vi "GUI PS Main Window.vi"() -> ()   [LabVIEW 2011]
uses:
  Types Definitions/Type GUI PS.ctl
  <vilib>/Platform/TimedLoop/XDataNode/timing_clust.ctl
  <vilib>/Platform/TimedLoop/XDataNode/nitl_modes.ctl
  <vilib>/Platform/TimedLoop/XDataNode/wakeup.ctl
  Types Definitions/Type Configuration Data (GUI to Controller).ctl
  Types Definitions/Type FOFB Parameters.ctl
  Types Definitions/Type Network Configuration.ctl
  Types Definitions/Type FA Configuration.ctl
  Types Definitions/Type Response Matrix Measurement Configuration.ctl
  Types Definitions/Type Correction Algorithm Configuration.ctl
  Types Definitions/Type Acquisition Network Configuration.ctl
  Types Definitions/Type Actuation Network Configuration.ctl
  Types Definitions/Type Configuration Change Acknowledge (Controller to GUI).ctl
  Types Definitions/Type TCP State.ctl
  <vilib>/Platform/TimedLoop/XDataNode/XDataNode.xnode
  <vilib>/Platform/TimedLoop/XDataNode/XDNodeRunTimeDep.lvlib
  LNLS Control VIs.lvlib
  Misc VIs.lvlib
  Type Definitions.lvlib
panel:
  out "PS Status":bool[](array[boolean])
  out "PS Setpoints":dbl[](array[numeric])
  in  "Step":dbl caption="Step (A)"
  in  "Configuration":dbl caption="Ajuste (A)"
  in  "Stop Test":bool
  out "Status":bool
  out "error out":errorcluster
  in  "PS Settings":bool
  in  "Initialize Test":bool
  # "FONTES CORRETORAS"
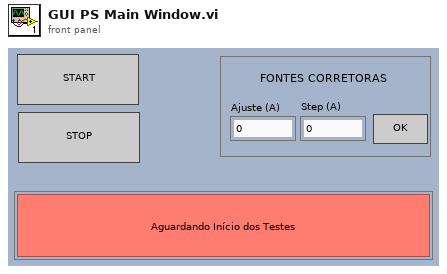
[diagram p1: front panel]
types:
  T1 = typedef "Type Definitions.lvlib/Type GUI PS.ctl" = cluster{"Change PS Value":refnum<notifier>, "Initialize/Stop RMM":refnum<notifier>, "Stop VI":refnum<notifier>, "Step Setpoint":refnum<notifier>}
  T2 = typedef "XDNodeRunTimeDep.lvlib/timing_clust.ctl" = cluster{"Expected End [f-1]":u64, "Actual End [f-1]":u64, "Finished Late? [f-1]":bool, "Expected End [i-1]":u64, "Actual End [i-1]":u64, "Finished Late? [i-1]":bool, "Expected Start [i]":u64, "Actual Start [i]":u64, "Expected Start [f]":u64, "Actual Start [f]":u64, "Source Name":string, "Structure Name":string, "Period":i64, "Deadline":i64, "Offset":i64, "Start":i64, "Priority":i32, "Timeout":i32, "Mode":T3, "Wakeup Reason":T4, "Error":errorcluster, "Source Type":string, "Secondary Source Type":string, "Global End Time":u64, "Global Start Time":u64, "Frame Duration":u64, "Iteration Duration":u64, "Assigned CPU":i32, "I/O Scan Engine Mode":u32}
  T3 = typedef "XDNodeRunTimeDep.lvlib/nitl_modes.ctl" = enum32{"No Change", "Process missed periods, maintain original phase", "Discard missed periods, maintain original phase", "Process missed periods, ignore original phase", "Discard missed periods, ignore original phase"}
  T4 = typedef "XDNodeRunTimeDep.lvlib/wakeup.ctl" = enum32{"Normal", "Aborted", "Asynchronous wakeup", "Timing source error", "Timed loop error", "Timeout"}
  T5 = enum16{"Wait Connection", "Read Data", "Write Data", "Close Connection", "Idle"}
  T6 = enum16{"Idle Mode", "Error Mode", "Manual Mode", "FOFB Mode", "RMM Mode"}
  T7 = cluster{"Operation Mode":enum16{"Idle Mode", "Error Mode", "Manual Mode", "FOFB Mode", "RMM Mode"}, "Correction Period (usec)":i32, "Beam Energy (MeV)":sgl, "Beam Current (mA)":sgl}
  T8 = typedef "Type Definitions.lvlib/Type LOCON_BIPOLAR_16BITS.ctl" = cluster{"priority":u8, "flag":u8, "analog value":u16, "status":u8}
  T9 = enum16{"Idle", "Wait Connection", "Read Data", "Process Data", "Write Data", "Close Connection"}
  T10 = typedef "Type Definitions.lvlib/Type Configuration Data (GUI to Controller).ctl" = cluster{"Update Controller Soft Configuration":bool[], "Request RT Execution Trace":string[], "Reference Orbit":dbl[], "Request Response Matrix Folder List":bool[], "Request FOFB Parameters":bool[], "FOFB Parameters":T11[]}
  T11 = typedef "Type Definitions.lvlib/Type FOFB Parameters.ctl" = cluster{"Network":T12, "Fast Acquisition":T13, "Response Matrix Measurement":T14, "Correction Algorithm":T15, "Acquisition Network":T16, "Actuation Network":T17}
  T12 = typedef "Type Definitions.lvlib/Type Network Configuration.ctl" = cluster{"FOFB Controller IP":string, "LNLS Control Network IP":string, "LNLS Control Network Power Supplies TCP Port":u16, "LNLS Control Network FOFB Configuration TCP Port":u16, "Data Server TCP Port":u16, "Monitoring Data TCP Port":u16, "Configuration GUI TCP Port":u16, "TCP Listening Timeout":i32}
  T13 = typedef "Type Definitions.lvlib/Type FA Configuration.ctl" = cluster{"Acquisition Period":u32, "Data Buffer Size":u32, "Monitoring Period":u32}
  T14 = typedef "Type Definitions.lvlib/Type Response Matrix Measurement Configuration.ctl" = cluster{"Step Amplitude":dbl, "Time Between Steps":u32, "Step Duration":u32, "Number of Averages":u32}
  T15 = typedef "Type Definitions.lvlib/Type Correction Algorithm Configuration.ctl" = cluster{"Correction Period":u32, "Reference Orbit Path":path, "Response Matrix Path":path, "Correction Matrix Path":path, "Horizontal Correction Factor":dbl, "Vertical Correction Factor":dbl, "Beam Current FOFB Threshold":dbl, "Decouple H-V":bool, "Use Additional BPM LPF":bool, "BPM LPF Cutoff":dbl}
  T16 = typedef "Type Definitions.lvlib/Type Acquisition Network Configuration.ctl" = cluster{"Chassis Name":string, "Variables":cluster{"Variable Name":string, "Matrix Order":u32, "Location":dbl, "Plane":enum8{"H", "V"}, "On Correction":bool}[]}[]
  T17 = typedef "Type Definitions.lvlib/Type Actuation Network Configuration.ctl" = cluster{"Chassis Name":string, "Variables":cluster{"Variable Name":string, "Matrix Order":u32, "RMM Step Factor":dbl, "Plane":enum8{"H", "V"}, "On Correction":bool, "Kc":dbl, "Ti":dbl, "Td":dbl}[]}[]
  T18 = typedef "Type Definitions.lvlib/Type Configuration Change Acknowledge (Controller to GUI).ctl" = cluster{"Request Response Matrix List Folder":string[], "FOFB Parameters":T11[]}
  T19 = typedef "Type Definitions.lvlib/Type TCP State.ctl" = enum16{"Idle", "Wait Connection", "Read Data", "Process Data", "Write Data", "Close Connection"}
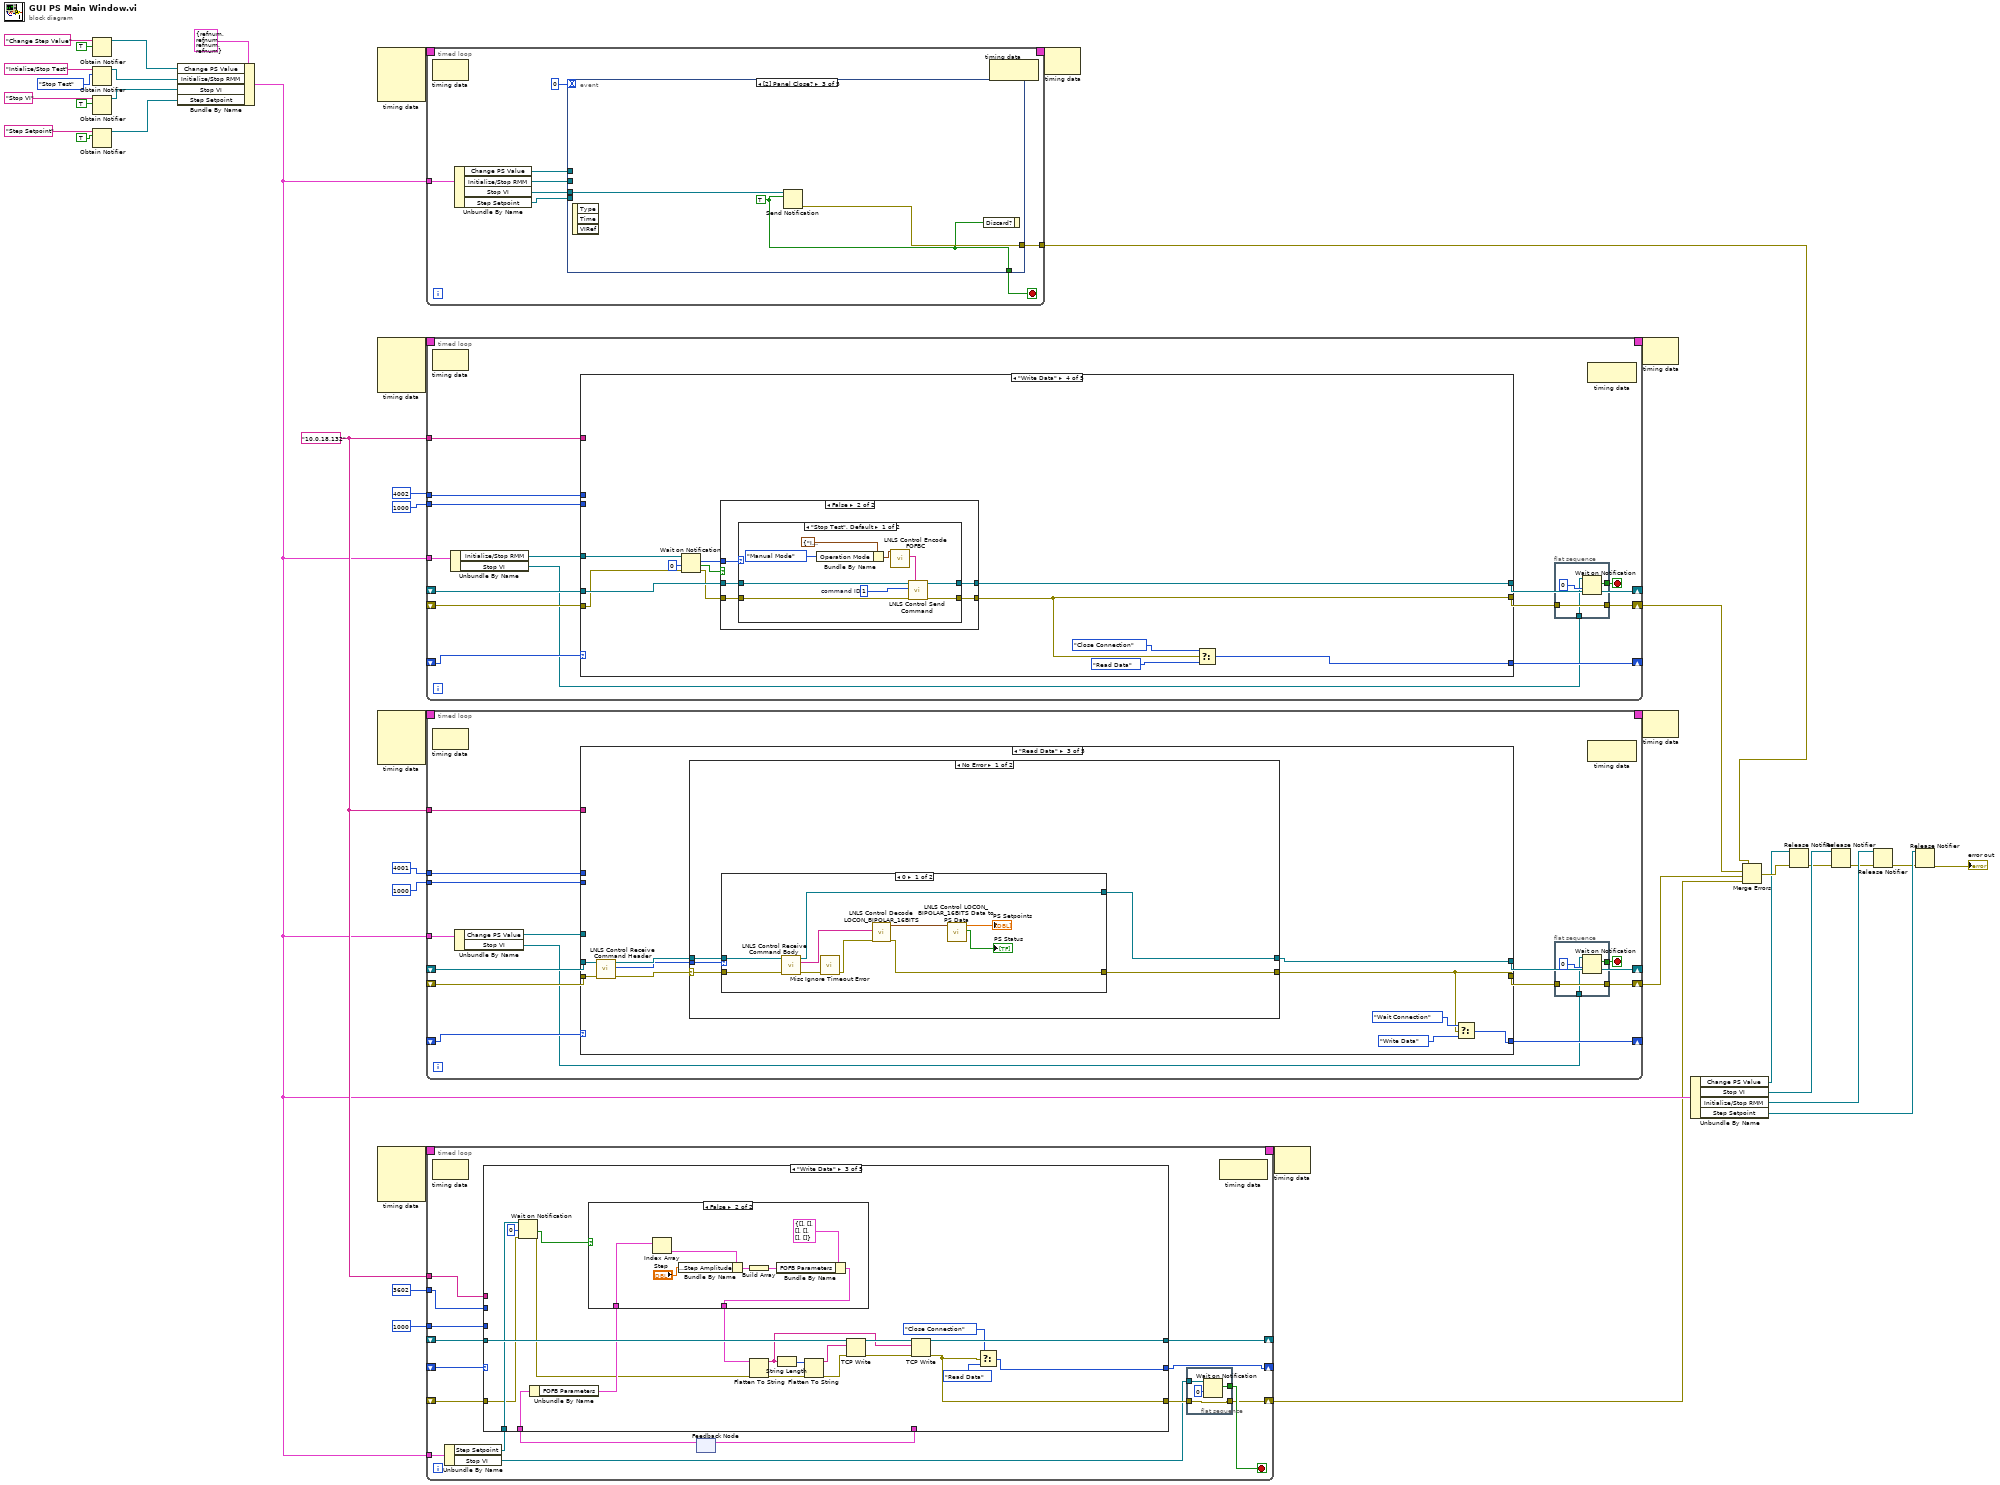
[diagram p0: block diagram]
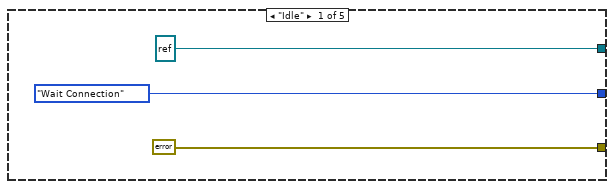
[diagram p2: hidden frame]
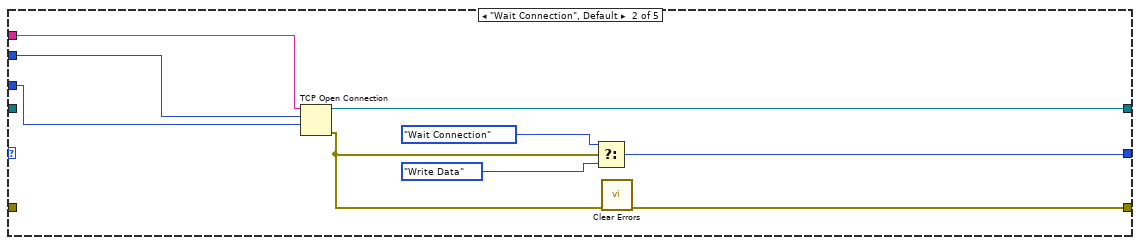
[diagram p3: hidden frame]
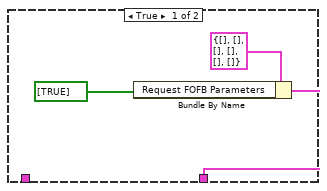
[diagram p4: hidden frame]
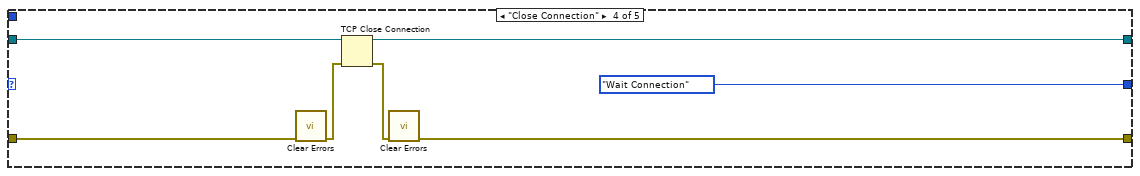
[diagram p5: hidden frame]
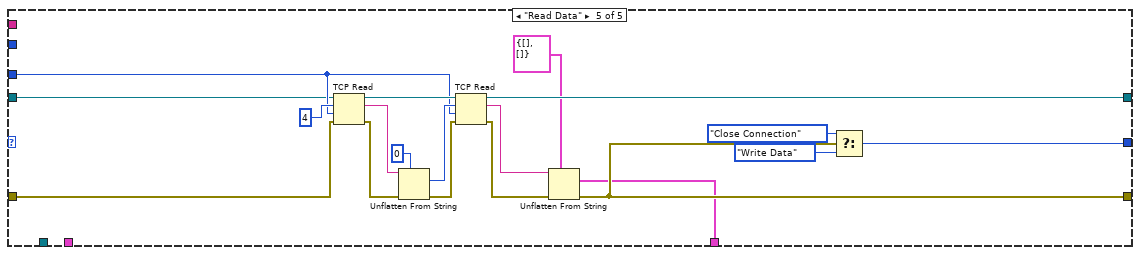
[diagram p6: hidden frame]
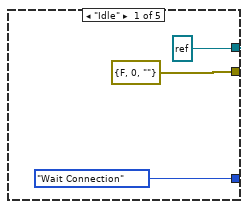
[diagram p7: hidden frame]
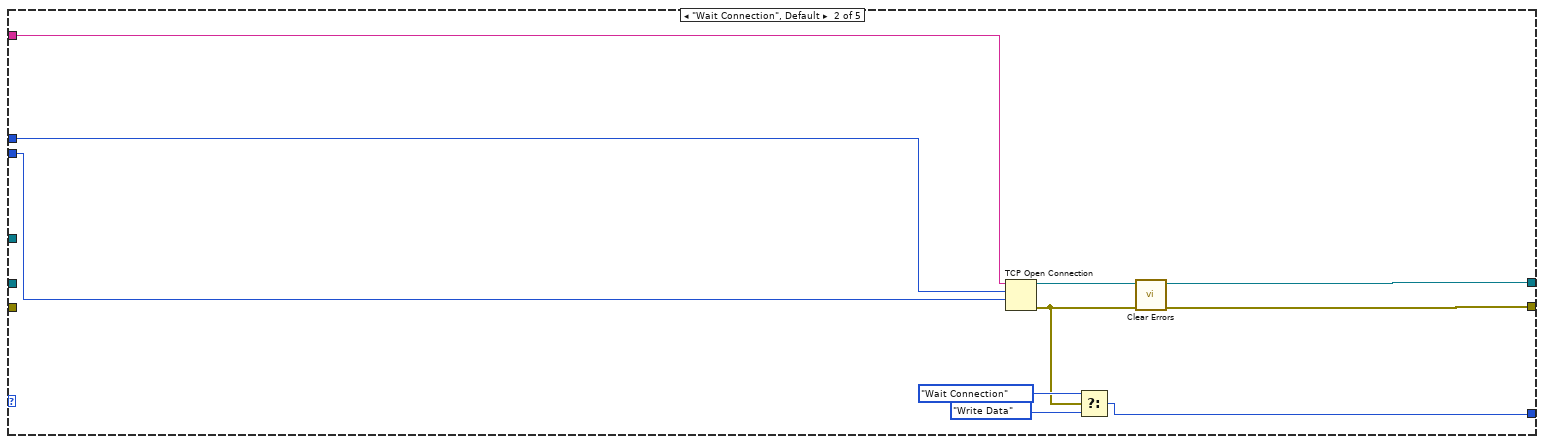
[diagram p8: hidden frame]
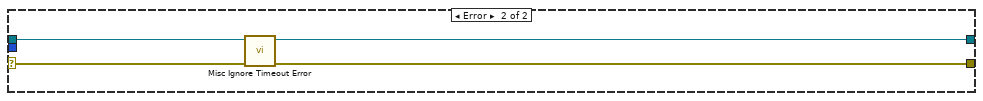
[diagram p10: hidden frame]
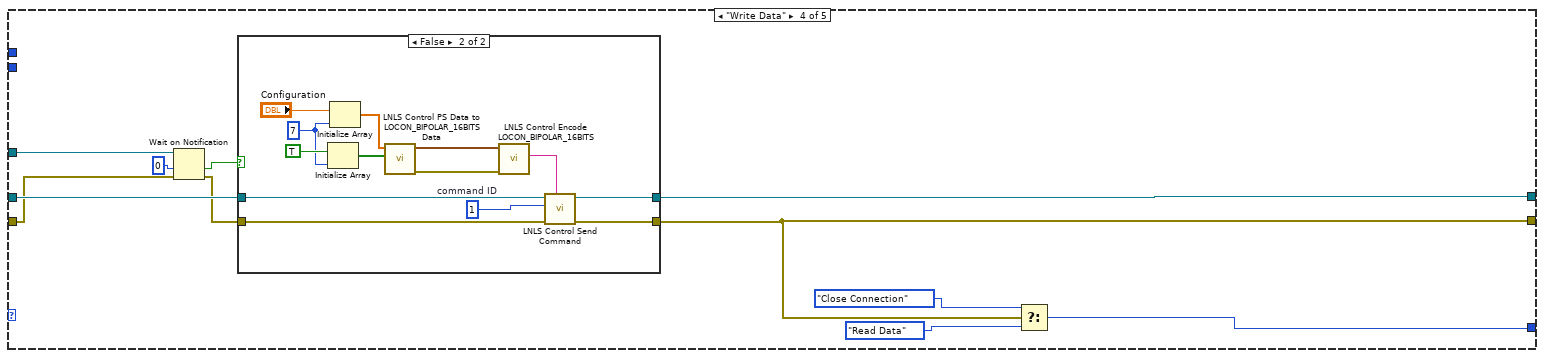
[diagram p11: hidden frame]
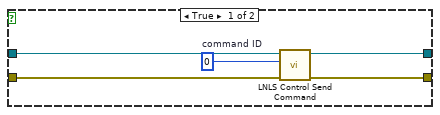
[diagram p12: hidden frame]
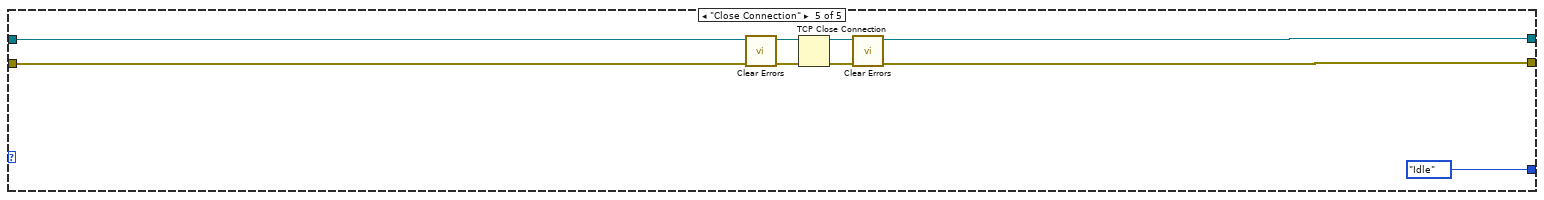
[diagram p13: hidden frame]
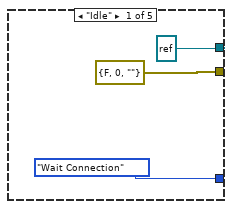
[diagram p14: hidden frame]
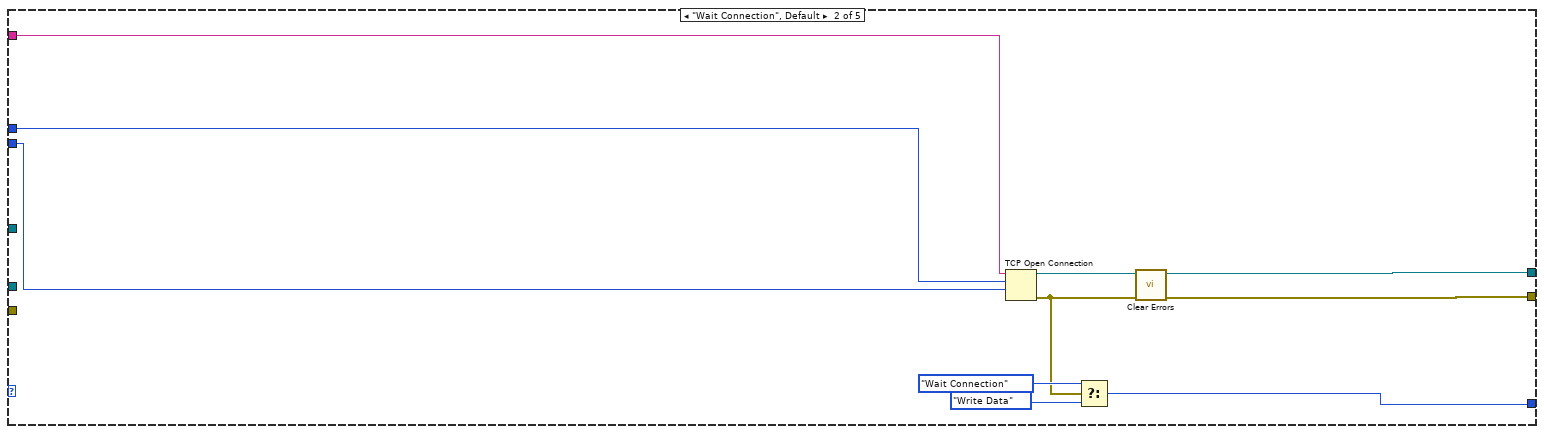
[diagram p15: hidden frame]
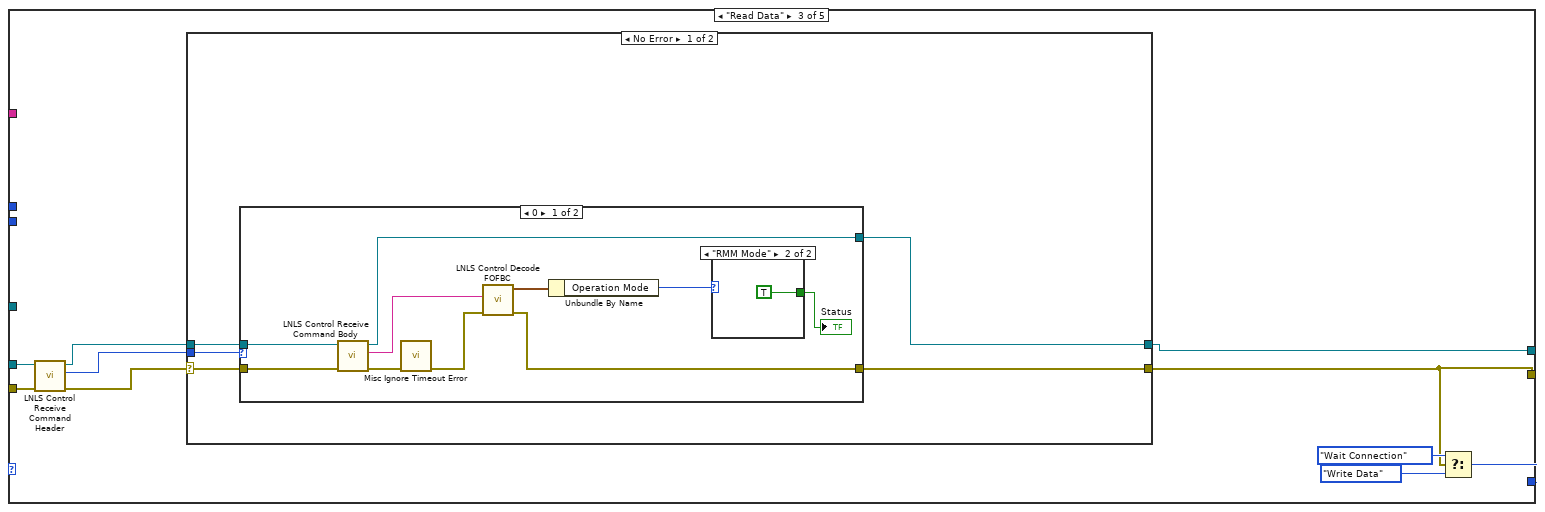
[diagram p16: hidden frame]
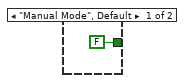
[diagram p17: hidden frame]
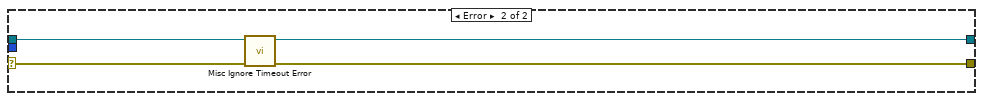
[diagram p19: hidden frame]
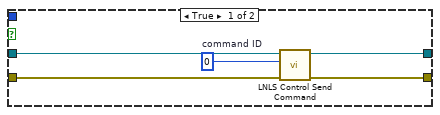
[diagram p20: hidden frame]
diagram:
  w12 = "10.0.18.132" ("address")
  n1 = Obtain Notifier(name (unnamed)="Change Step Value", notification data type=TRUE) -> (notifier out=w33:refnum<notifier>)  [unwired: 2 in, 2 out]
  n2 = Obtain Notifier(name (unnamed)="Intialize/Stop Test", notification data type=enum16{"Initialize Test", "Stop Test"}."Stop Test") -> (notifier out=w21:refnum<notifier>)  [unwired: 2 in, 2 out]
  n3 = Obtain Notifier(name (unnamed)="Stop VI", notification data type=TRUE) -> (notifier out=w32:refnum<notifier>)  [unwired: 2 in, 2 out]
  n4 = Obtain Notifier(name (unnamed)="Step Setpoint", notification data type=TRUE) -> (notifier out=w7:refnum<notifier>)  [unwired: 2 in, 2 out]
  n5 = Bundle By Name(cluster=T1 {"Change PS Value"=refnum, "Initialize/Stop RMM"=refnum, "Stop VI"=refnum, "Step Setpoint"=refnum} ("GUI PS"), "Change PS Value"=w33, "Initialize/Stop RMM"=w21, "Stop VI"=w32, "Step Setpoint"=w7) -> (w6:T1)
  n6 = node-c288() -> (w37:T2)  [unwired: 4 in]
  n7 = node-c288() -> (w26:T2)  [unwired: 4 in]
  n8 = node-c288() -> (w18:T2)  [unwired: 4 in]
  n9 = node-c288() -> (w14:T2)  [unwired: 4 in]
  n10 = timed-loop {
    timing: w37 -> [_]
    timing-out: [_] -> w36
    tunnel: [w48] -> w35
    tunnel: w6 -> [w47]
    stop <- w50 stop-if-true
    n11 = node-c288() -> ()  [unwired: 1 in, 1 out]
    n12 = Unbundle By Name(w47) -> ("Change PS Value"=w46:refnum<notifier>, "Initialize/Stop RMM"=w45:refnum<notifier>, "Stop VI"=w44:refnum<notifier>, "Step Setpoint"=w43:refnum<notifier>)
    n13 = event shown="[2] Panel Close?" {
      selector: _ -> [_ _ _ _ _]
      dyn-events: _ -> [_ _ _ _ _]
      timeout: 0 -> [_ _ _ _ _]
      tunnel: [_ _ w55 _ _] -> w50
      tunnel: [_ _ w57 _ _] -> w48
      tunnel: w46 -> [_ _ _ _ w64]
      tunnel: w45 -> [_ w52 _ w59 _]
      tunnel: w44 -> [_ _ w56 _ _]
      tunnel: w43 -> [_ _ _ _ w62]
      event Timeout {
        n14 = event-data() -> ()  [unwired: 1 in, 2 out]
      }
      event "Stop Test": Value Change {
        n15 = event-data() -> ("NewVal"=w51:bool)  [unwired: 1 in, 4 out]
        n16 = case shown="True" w51 {
          tunnel: w52 -> [_ w54]
          frame False {
          }
          frame True {
            n17 = Send Notification(notification=enum16{"Initialize Test", "Stop Test"}."Stop Test", notifier=w54) -> ()  [unwired: 1 in, 2 out]
          }
        }
      }
      event Panel Close? {
        w55 = TRUE
        n18 = event-data() -> ()  [unwired: 1 in, 3 out]
        n19 = Send Notification(notification=w55, notifier=w56) -> (error out=w57:errorcluster)  [unwired: 1 in, 1 out]
        n20 = event-data("Discard?"=w55) -> ()  [unwired: 1 in, 1 out]
      }
      event "Initialize Test": Value Change {
        n21 = event-data() -> ("NewVal"=w58:bool)  [unwired: 1 in, 4 out]
        n22 = case shown="True" w58 {
          tunnel: w59 -> [_ w61]
          frame False {
          }
          frame True {
            n23 = Send Notification(notification=enum16{"Initialize Test", "Stop Test"}."Initialize Test", notifier=w61) -> ()  [unwired: 1 in, 2 out]
          }
        }
      }
      event "PS Settings": Value Change {
        n24 = event-data() -> ("NewVal"=w63:bool)  [unwired: 1 in, 4 out]
        n25 = case shown="True" w63 {
          selector: w63 -> [_ w65]
          tunnel: w64 -> [_ w67]
          tunnel: w62 -> [_ w66]
          frame False {
          }
          frame True {
            n26 = Send Notification(notification=w65, notifier=w67) -> ()  [unwired: 1 in, 2 out]
            n27 = Send Notification(notification=w65, notifier=w66) -> ()  [unwired: 1 in, 2 out]
          }
        }
      }
    }
    n28 = node-c288() -> ()  [unwired: 1 in, 1 out]
  }
  n29 = timed-loop {
    shift-right: [w81] -> _
    shift-left: _ -> [w83]
    shift-right: [w82] -> _
    shift-left: _ -> [w80]
    shift-right: [w74] -> w20
    shift-left: _ -> [w79]
    tunnel: u16 4002 ("remote port or service name") -> [w78]
    tunnel: 1000 ("timeout ms (60000)") -> [w76]
    timing: w26 -> [_]
    timing-out: [_] -> w25
    tunnel: w12 -> [w73]
    tunnel: w6 -> [w72]
    stop <- w77 stop-if-true
    n30 = node-c288() -> ()  [unwired: 1 in, 1 out]
    n31 = Unbundle By Name(w72) -> ("Initialize/Stop RMM"=w70:refnum<notifier>, "Stop VI"=w71:refnum<notifier>)
    n32 = case shown="\"Write Data\"" w83 {
      tunnel: [refnum<k5> refnum ("connection ID") w94 w107 w137 w175] -> w82
      tunnel: [errorcluster {"status"=FALSE, "code"=0, "source"=""} ("error out") w92 w99 w139 w172] -> w75
      tunnel: [T5."Wait Connection" w97 w106 w140 T5."Idle"] -> w81
      tunnel: w80 -> [_ _ w104 w138 w176]
      tunnel: w79 -> [_ _ w105 w133 w170]
      tunnel: w78 -> [_ w91 _ _ _]
      tunnel: w76 -> [_ w90 _ _ _]
      tunnel: w73 -> [_ w89 _ _ _]
      tunnel: w70 -> [_ _ _ w136 _]
      frame "Idle" {
      }
      frame "Wait Connection", Default {
        n33 = TCP Open Connection(address=w89, remote port or service name=w91, timeout ms (60000)=w90) -> (connection ID=w94:refnum<k5>, error out=w93:errorcluster)  [unwired: 2 in]
        n34 = Select(t=T5."Wait Connection", s=w93, f=T5."Write Data") -> (s? t:f=w97:T5)
        n35 = call <vilib>:"Clear Errors.vi"("error in (no error)"=w93) -> ("error out"=w92:errorcluster)  [unwired: 6 in]
      }
      frame "Read Data" {
        n36 = call "LNLS Control Receive Command Header.vi"("error in (no error)"=w105, "connection ID"=w104) -> ("error out"=w101:errorcluster, "command ID"=w98:u8, "connection ID out"=w103:refnum<k5>)  [unwired: 7 in]
        n37 = case shown="No Error" w101 {
          selector: w101 -> [w111 w128]
          tunnel: [w110 w129] -> w107
          tunnel: [w108 w127] -> w99
          tunnel: w103 -> [w112 w129]
          tunnel: w98 -> [w109 _]
          frame No Error {
            n38 = case shown="0" w109 {
              tunnel: w112 -> [w122 w126]
              tunnel: w111 -> [w121 w125]
              tunnel: [w120 w126] -> w110
              tunnel: [w119 w125] -> w108
              frame 0 {
                n39 = call "LNLS Control Receive Command Body.vi"("error in (no error)"=w121, "connection ID"=w122) -> ("error out"=w118:errorcluster, "command body"=w116:string, "connection ID out"=w120:refnum<k5>)  [unwired: 6 in, 1 out]
                n40 = call "Misc Ignore Timeout Error.vi"("error in (no error)"=w118) -> ("error out"=w117:errorcluster)  [unwired: 10 in]
                n41 = call "LNLS Control Decode FOFBC.vi"("error in (no error)"=w117, "command body"=w116) -> ("error out"=w119:errorcluster, "LNLS Control FOFB Configuration"=w115:T7)  [unwired: 8 in]
                n42 = Unbundle By Name(w115) -> ("Operation Mode"=w114:T6)
                n43 = case shown="\"RMM Mode\"" w114 {
                  tunnel: [FALSE TRUE] -> w113
                  frame "Manual Mode", Default {
                  }
                  frame "RMM Mode" {
                  }
                }
                "Status" <- w113
              }
              frame 1, Default {
              }
            }
          }
          frame Error {
            n44 = call "Misc Ignore Timeout Error.vi"("error in (no error)"=w128) -> ("error out"=w127:errorcluster)  [unwired: 10 in]
          }
        }
        n45 = Select(t=T5."Wait Connection", s=w99, f=T5."Write Data") -> (s? t:f=w106:T5)
      }
      frame "Write Data" {
        n46 = Wait on Notification(notifier=w136, timeout in ms (-1)=0, error in (no error)=w133) -> (notification=w135:enum16{"Initialize Test", "Stop Test"}, timed out?=w130:bool, error out=w132:errorcluster)  [unwired: 1 in, 1 out]
        n47 = case shown="False" w130 {
          tunnel: [w144 w151] -> w139
          tunnel: w138 -> [w143 w150]
          tunnel: [w142 w149] -> w137
          tunnel: w135 -> [_ w148]
          tunnel: w132 -> [w145 w147]
          frame True {
            w146 = u8 0  # command ID
            n48 = call "LNLS Control Send Command.vi"("error in (no error)"=w145, "command ID"=w146, "connection ID"=w143) -> ("error out"=w144:errorcluster, "connection ID out"=w142:refnum<k5>)  [unwired: 7 in]
          }
          frame False {
            n49 = case shown="\"Stop Test\", Default" w148 {
              tunnel: w147 -> [w160 w169]
              tunnel: [w159 w168] -> w151
              tunnel: w150 -> [w158 w167]
              tunnel: [w157 w166] -> w149
              frame "Stop Test", Default {
                w156 = u8 1  # command ID
                n50 = Bundle By Name(cluster=T7 {"Operation Mode"=enum."Idle Mode", "Correction Period (usec)"=0, "Beam Energy (MeV)"=0.0, "Beam Current (mA)"=0.0} ("LNLS Control FOFB Configuration"), "Operation Mode"=T6."Manual Mode") -> (w152:T7)
                n51 = call "LNLS Control Encode FOFBC.vi"("LNLS Control FOFB Configuration"=w152) -> ("command body"=w155:string)  [unwired: 9 in, 1 out]
                n52 = call "LNLS Control Send Command.vi"("command body"=w155, "error in (no error)"=w160, "command ID"=w156, "connection ID"=w158) -> ("error out"=w159:errorcluster, "connection ID out"=w157:refnum<k5>)  [unwired: 6 in]
              }
              frame "Initialize Test" {
                w165 = u8 1  # command ID
                n53 = Bundle By Name(cluster=T7 {"Operation Mode"=enum."Idle Mode", "Correction Period (usec)"=0, "Beam Energy (MeV)"=0.0, "Beam Current (mA)"=0.0} ("LNLS Control FOFB Configuration"), "Operation Mode"=T6."RMM Mode") -> (w161:T7)
                n54 = call "LNLS Control Encode FOFBC.vi"("LNLS Control FOFB Configuration"=w161) -> ("command body"=w164:string)  [unwired: 9 in, 1 out]
                n55 = call "LNLS Control Send Command.vi"("command body"=w164, "error in (no error)"=w169, "command ID"=w165, "connection ID"=w167) -> ("error out"=w168:errorcluster, "connection ID out"=w166:refnum<k5>)  [unwired: 6 in]
              }
            }
          }
        }
        n56 = Select(t=T5."Close Connection", s=w139, f=T5."Read Data") -> (s? t:f=w140:T5)
      }
      frame "Close Connection" {
        n57 = call <vilib>:"Clear Errors.vi"("error in (no error)"=w170) -> ("error out"=w171:errorcluster)  [unwired: 6 in]
        n58 = TCP Close Connection(connection ID=w176, error in (no error)=w171) -> (connection ID out=w175:refnum<k5>, error out=w173:errorcluster)  [unwired: 1 in]
        n59 = call <vilib>:"Clear Errors.vi"("error in (no error)"=w173) -> ("error out"=w172:errorcluster)  [unwired: 6 in]
      }
    }
    n60 = flat-sequence {
      tunnel: [w179] -> w77
      tunnel: w75 -> [w178]
      tunnel: [w178] -> w74
      tunnel: w71 -> [w177]
      frame #0 {
        n61 = Wait on Notification(notifier=w177, timeout in ms (-1)=0) -> (notification=w179:bool)  [unwired: 2 in, 3 out]
      }
    }
    n62 = node-c288() -> ()  [unwired: 1 in, 1 out]
  }
  n63 = timed-loop {
    shift-right: [w192] -> _
    shift-left: _ -> [w194]
    shift-right: [w193] -> _
    shift-left: _ -> [w191]
    shift-right: [w185] -> w19
    shift-left: _ -> [w190]
    tunnel: u16 4001 ("remote port or service name") -> [w189]
    tunnel: 1000 ("timeout ms (60000)") -> [w187]
    timing: w18 -> [_]
    timing-out: [_] -> w17
    tunnel: w12 -> [w184]
    tunnel: w6 -> [w183]
    stop <- w188 stop-if-true
    n64 = node-c288() -> ()  [unwired: 1 in, 1 out]
    n65 = Unbundle By Name(w183) -> ("Change PS Value"=w181:refnum<notifier>, "Stop VI"=w182:refnum<notifier>)
    n66 = case shown="\"Read Data\"" w194 {
      tunnel: [refnum<k5> refnum ("connection ID") w205 w218 w245 w273] -> w193
      tunnel: [errorcluster {"status"=FALSE, "code"=0, "source"=""} ("error out") w203 w210 w247 w270] -> w186
      tunnel: [T5."Wait Connection" w208 w217 w248 T5."Idle"] -> w192
      tunnel: w191 -> [_ _ w215 w246 w274]
      tunnel: w190 -> [_ _ w216 w242 w268]
      tunnel: w189 -> [_ w202 _ _ _]
      tunnel: w187 -> [_ w201 _ _ _]
      tunnel: w184 -> [_ w200 _ _ _]
      tunnel: w181 -> [_ _ _ w244 _]
      frame "Idle" {
      }
      frame "Wait Connection", Default {
        n67 = TCP Open Connection(address=w200, remote port or service name=w202, timeout ms (60000)=w201) -> (connection ID=w205:refnum<k5>, error out=w204:errorcluster)  [unwired: 2 in]
        n68 = Select(t=T5."Wait Connection", s=w204, f=T5."Write Data") -> (s? t:f=w208:T5)
        n69 = call <vilib>:"Clear Errors.vi"("error in (no error)"=w204) -> ("error out"=w203:errorcluster)  [unwired: 6 in]
      }
      frame "Read Data" {
        n70 = call "LNLS Control Receive Command Header.vi"("error in (no error)"=w216, "connection ID"=w215) -> ("error out"=w212:errorcluster, "command ID"=w209:u8, "connection ID out"=w214:refnum<k5>)  [unwired: 7 in]
        n71 = case shown="No Error" w212 {
          selector: w212 -> [w222 w237]
          tunnel: [w221 w238] -> w218
          tunnel: [w219 w236] -> w210
          tunnel: w214 -> [w223 w238]
          tunnel: w209 -> [w220 _]
          frame No Error {
            n72 = case shown="0" w220 {
              tunnel: w223 -> [w233 w235]
              tunnel: w222 -> [w232 w234]
              tunnel: [w231 w235] -> w221
              tunnel: [w227 w234] -> w219
              frame 0 {
                n73 = call "LNLS Control Receive Command Body.vi"("error in (no error)"=w232, "connection ID"=w233) -> ("error out"=w230:errorcluster, "command body"=w229:string, "connection ID out"=w231:refnum<k5>)  [unwired: 6 in, 1 out]
                n74 = call "Misc Ignore Timeout Error.vi"("error in (no error)"=w230) -> ("error out"=w228:errorcluster)  [unwired: 10 in]
                n75 = call "LNLS Control Decode LOCON_BIPOLAR_16BITS.vi"("error in (no error)"=w228, "command body"=w229) -> ("error out"=w227:errorcluster, "LOCON data"=w226:T8[])  [unwired: 6 in]
                n76 = call "LNLS Control LOCON_BIPOLAR_16BITS Data to PS Data.vi"("PS Setpoints LOCON Data"=w226) -> ("PS Status"=→"PS Status":bool[], "PS Setpoints"=→"PS Setpoints":dbl[])  [unwired: 8 in, 1 out]
              }
              frame 1, Default {
              }
            }
          }
          frame Error {
            n77 = call "Misc Ignore Timeout Error.vi"("error in (no error)"=w237) -> ("error out"=w236:errorcluster)  [unwired: 10 in]
          }
        }
        n78 = Select(t=T5."Wait Connection", s=w210, f=T5."Write Data") -> (s? t:f=w217:T5)
      }
      frame "Write Data" {
        n79 = Wait on Notification(notifier=w244, timeout in ms (-1)=0, error in (no error)=w242) -> (timed out?=w239:bool, error out=w241:errorcluster)  [unwired: 1 in, 2 out]
        n80 = case shown="False" w239 {
          tunnel: [w252 w267] -> w247
          tunnel: w246 -> [w251 w266]
          tunnel: [w250 w265] -> w245
          tunnel: w241 -> [w253 w264]
          frame True {
            w254 = u8 0  # command ID
            n81 = call "LNLS Control Send Command.vi"("error in (no error)"=w253, "command ID"=w254, "connection ID"=w251) -> ("error out"=w252:errorcluster, "connection ID out"=w250:refnum<k5>)  [unwired: 7 in]
          }
          frame False {
            w256 = 7 ("dimension size")
            w263 = u8 1  # command ID
            n82 = Initialize Array(TRUE, w256) -> (w255:bool[])
            n83 = Initialize Array("Configuration", w256) -> (w258:dbl[])
            n84 = call "LNLS Control PS Data to LOCON_BIPOLAR_16BITS Data.vi"("PS Status"=w255, "PS Readings/Setpoints"=w258) -> ("error out"=w260:errorcluster, "PS Readings/Setpoints LOCON Data"=w262:T8[])  [unwired: 8 in]
            n85 = call "LNLS Control Encode LOCON_BIPOLAR_16BITS.vi"("error in (no error)"=w260, "LOCON Data"=w262) -> ("command body"=w261:string)  [unwired: 8 in, 1 out]
            n86 = call "LNLS Control Send Command.vi"("command body"=w261, "error in (no error)"=w264, "command ID"=w263, "connection ID"=w266) -> ("error out"=w267:errorcluster, "connection ID out"=w265:refnum<k5>)  [unwired: 6 in]
          }
        }
        n87 = Select(t=T5."Close Connection", s=w247, f=T5."Read Data") -> (s? t:f=w248:T5)
      }
      frame "Close Connection" {
        n88 = call <vilib>:"Clear Errors.vi"("error in (no error)"=w268) -> ("error out"=w269:errorcluster)  [unwired: 6 in]
        n89 = TCP Close Connection(connection ID=w274, error in (no error)=w269) -> (connection ID out=w273:refnum<k5>, error out=w271:errorcluster)  [unwired: 1 in]
        n90 = call <vilib>:"Clear Errors.vi"("error in (no error)"=w271) -> ("error out"=w270:errorcluster)  [unwired: 6 in]
      }
    }
    n91 = flat-sequence {
      tunnel: [w277] -> w188
      tunnel: w186 -> [w276]
      tunnel: [w276] -> w185
      tunnel: w182 -> [w275]
      frame #0 {
        n92 = Wait on Notification(notifier=w275, timeout in ms (-1)=0) -> (notification=w277:bool)  [unwired: 2 in, 3 out]
      }
    }
    n93 = node-c288() -> ()  [unwired: 1 in, 1 out]
  }
  n94 = timed-loop {
    timing: w14 -> [_]
    timing-out: [_] -> w13
    shift-right: [w280] -> _
    shift-left: _ -> [w294]
    shift-right: [w292] -> _
    shift-left: _ -> [w293]
    tunnel: w12 -> [w291]
    tunnel: u16 3602 ("Configuration GUI TCP Port") -> [w290]
    tunnel: 1000 ("TCP Listening Timeout") -> [w289]
    tunnel: w6 -> [w287]
    shift-right: [w284] -> w2
    shift-left: _ -> [w285]
    stop <- w286 stop-if-true
    n95 = node-c288() -> ()  [unwired: 1 in, 1 out]
    n96 = Unbundle By Name(w287) -> ("Step Setpoint"=w279:refnum<notifier>, "Stop VI"=w283:refnum<notifier>)
    n97 = feedback #1() -> (w281:T18)  [unwired: 1 in]
    n98 = case shown="\"Write Data\"" w294 {
      tunnel: [refnum<k5> refnum ("connection ID") w306 w331 w348 w353] -> w292
      tunnel: [T9."Wait Connection" ("f") w310 w314 T9."Wait Connection" ("f") w351] -> w280
      tunnel: [errorcluster {"status"=FALSE, "code"=0, "source"=""} ("error out") w309 w317 w347 w352] -> w288
      tunnel: w285 -> [_ _ w313 w342 w354]
      tunnel: w293 -> [_ _ w330 w343 w355]
      tunnel: w291 -> [_ w304 _ _ _]
      tunnel: w290 -> [_ w303 _ _ _]
      tunnel: w289 -> [_ w302 _ _ w356]
      tunnel: w279 -> [_ _ w321 _ _]
      tunnel: [_ _ _ _ w349] -> w282
      tunnel: w281 -> [_ _ w320 _ _]
      frame "Idle" {
      }
      frame "Wait Connection", Default {
        n99 = TCP Open Connection(address=w304, remote port or service name=w303, timeout ms (60000)=w302) -> (connection ID=w306:refnum<k5>, error out=w305:errorcluster)  [unwired: 2 in]
        n100 = Select(t=T9."Wait Connection" ("f"), s=w305, f=T9."Write Data") -> (s? t:f=w310:T9)
        n101 = call <vilib>:"Clear Errors.vi"("error in (no error)"=w305) -> ("error out"=w309:errorcluster)  [unwired: 6 out]
      }
      frame "Write Data" {
        n102 = Wait on Notification(notifier=w321, timeout in ms (-1)=0, error in (no error)=w313) -> (timed out?=w318:bool, error out=w312:errorcluster)  [unwired: 1 in, 2 out]
        n103 = Unbundle By Name(w320) -> ("FOFB Parameters"=w319:T11[])
        n104 = case shown="False" w318 {
          tunnel: [w332 w341] -> w322
          tunnel: w319 -> [_ w339]
          frame True {
            n105 = Bundle By Name(cluster=T10 {"Update Controller Soft Configuration"=[], "Request RT Execution Trace"=[], "Reference Orbit"=[], "Request Response Matrix Folder List"=[], "Request FOFB Parameters"=[], "FOFB Parameters"=[]} ("Configuration Data (GUI to Controller)"), "Request FOFB Parameters"=bool[] [TRUE] ("Request Folder List")) -> (w332:T10)
          }
          frame False {
            n106 = Index Array(array=w339) -> (element=w338:T11)  [unwired: 1 in]
            n107 = Bundle By Name(cluster=w338, "Response Matrix Measurement.Step Amplitude"="Step") -> (w336:T11)
            n108 = Build Array(w336) -> (w335:T11[])
            n109 = Bundle By Name(cluster=T10 {"Update Controller Soft Configuration"=[], "Request RT Execution Trace"=[], "Reference Orbit"=[], "Request Response Matrix Folder List"=[], "Request FOFB Parameters"=[], "FOFB Parameters"=[]} ("Configuration Data (GUI to Controller)"), "FOFB Parameters"=w335) -> (w341:T10)
          }
        }
        n110 = Flatten To String(anything=w322, error in (no error)=w312) -> (data string=w325:string, error out=w324:errorcluster)  [unwired: 2 in, 1 out]
        n111 = String Length(string=w325) -> (length=w327:i32)
        n112 = Flatten To String(anything=w327, error in (no error)=w324) -> (data string=w326:string, error out=w323:errorcluster)  [unwired: 2 in, 1 out]
        n113 = TCP Write(connection ID=w330, data in=w326, error in (no error)=w323) -> (connection ID out=w329:refnum<k5>, error out=w328:errorcluster)  [unwired: 2 out]
        n114 = TCP Write(connection ID=w329, data in=w325, error in (no error)=w328) -> (connection ID out=w331:refnum<k5>, error out=w317:errorcluster)  [unwired: 2 out]
        n115 = Select(t=T9."Close Connection" ("f"), s=w317, f=T9."Read Data") -> (s? t:f=w314:T9)
      }
      frame "Close Connection" {
        n116 = call <vilib>:"Clear Errors.vi"("error in (no error)"=w342) -> ("error out"=w346:errorcluster)  [unwired: 6 in]
        n117 = TCP Close Connection(connection ID=w343, error in (no error)=w346) -> (connection ID out=w348:refnum<k5>, error out=w345:errorcluster)  [unwired: 1 in]
        n118 = call <vilib>:"Clear Errors.vi"("error in (no error)"=w345) -> ("error out"=w347:errorcluster)  [unwired: 6 in]
      }
      frame "Read Data" {
        n119 = TCP Read(connection ID=w355, bytes to read=4, error in (no error)=w354, 9:w356) -> (connection ID out=w367:refnum<k5>, data out=w365:string, error out=w358:errorcluster)  [unwired: 1 in]
        n120 = Unflatten From String(type=0 ("bytes to read"), binary string=w365, error in (no error)=w358) -> (value=w363:i32, error out=w359:errorcluster)  [unwired: 2 in, 1 out]
        n121 = TCP Read(connection ID=w367, bytes to read=w363, error in (no error)=w359, 9:w356) -> (connection ID out=w353:refnum<k5>, data out=w362:string, error out=w357:errorcluster)  [unwired: 1 in]
        n122 = Unflatten From String(type=T18 {"Request Response Matrix List Folder"=[], "FOFB Parameters"=[]} ("Configuration Change Acknowledge (Controller to GUI)"), binary string=w362, error in (no error)=w357) -> (value=w349:T18, error out=w352:errorcluster)  [unwired: 2 in, 1 out]
        n123 = Select(t=Type_TCP_State."Close Connection" ("f"), s=w352, f=Type_TCP_State."Write Data") -> (s? t:f=w351:T19)
      }
    }
    n124 = feedback-in #1(w282) -> ()
    n125 = flat-sequence {
      tunnel: [w298] -> w286
      tunnel: w288 -> [w296]
      tunnel: [w296] -> w284
      tunnel: w283 -> [w295]
      frame #0 {
        n126 = Wait on Notification(notifier=w295, timeout in ms (-1)=0) -> (notification=w298:bool)  [unwired: 2 in, 3 out]
      }
    }
    n127 = node-c288() -> ()  [unwired: 1 in, 1 out]
  }
  n128 = node-c288(w36) -> ()  [unwired: 1 out]
  n129 = node-c288(w13) -> ()  [unwired: 1 out]
  n130 = node-c288(w25) -> ()  [unwired: 1 out]
  n131 = node-c288(w17) -> ()  [unwired: 1 out]
  n132 = Unbundle By Name(w6) -> ("Change PS Value"=w31:refnum<notifier>, "Stop VI"=w30:refnum<notifier>, "Initialize/Stop RMM"=w29:refnum<notifier>, "Step Setpoint"=w5:refnum<notifier>)
  n133 = Merge Errors(w35, w20, w19, w2) -> (w34:errorcluster)
  n134 = Release Notifier(notifier=w31, error in (no error)=w34) -> (error out=w28:errorcluster)  [unwired: 1 in, 2 out]
  n135 = Release Notifier(notifier=w30, error in (no error)=w28) -> (error out=w27:errorcluster)  [unwired: 1 in, 2 out]
  n136 = Release Notifier(notifier=w29, error in (no error)=w27) -> (error out=w4:errorcluster)  [unwired: 1 in, 2 out]
  n137 = Release Notifier(notifier=w5, error in (no error)=w4) -> (error out=→"error out":errorcluster)  [unwired: 1 in, 2 out]
